vi "Scale and Checksum.vi"(0 "Raw Data":bool[](array[boolean])=[FALSE, FALSE, FALSE, FALSE, FALSE, FALSE, FALSE, FALSE, FALSE, FALSE, FALSE, FALSE, FALSE, FALSE, FALSE, FALSE, FALSE, FALSE, FALSE, FALSE, FALSE, FALSE, FALSE, FALSE, FALSE, FALSE, FALSE, FALSE, FALSE, FALSE, FALSE, FALSE, FALSE, FALSE, FALSE, FALSE, FALSE, FALSE, FALSE, FALSE]) -> (4 "Temperature (°C)":fxp<+,16,7> format="%.12g", 8 "Humidity (%)":fxp<+/-,18,8> format="%.13g", 15 "Valid?":bool)   [LabVIEW 2016, in "DHT22 (FPGA).lvlib"]
uses:
  DHT22 (FPGA).lvlib
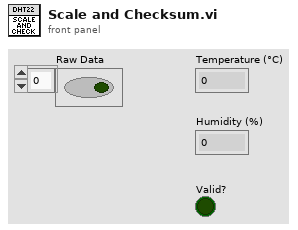
[diagram p1: front panel]
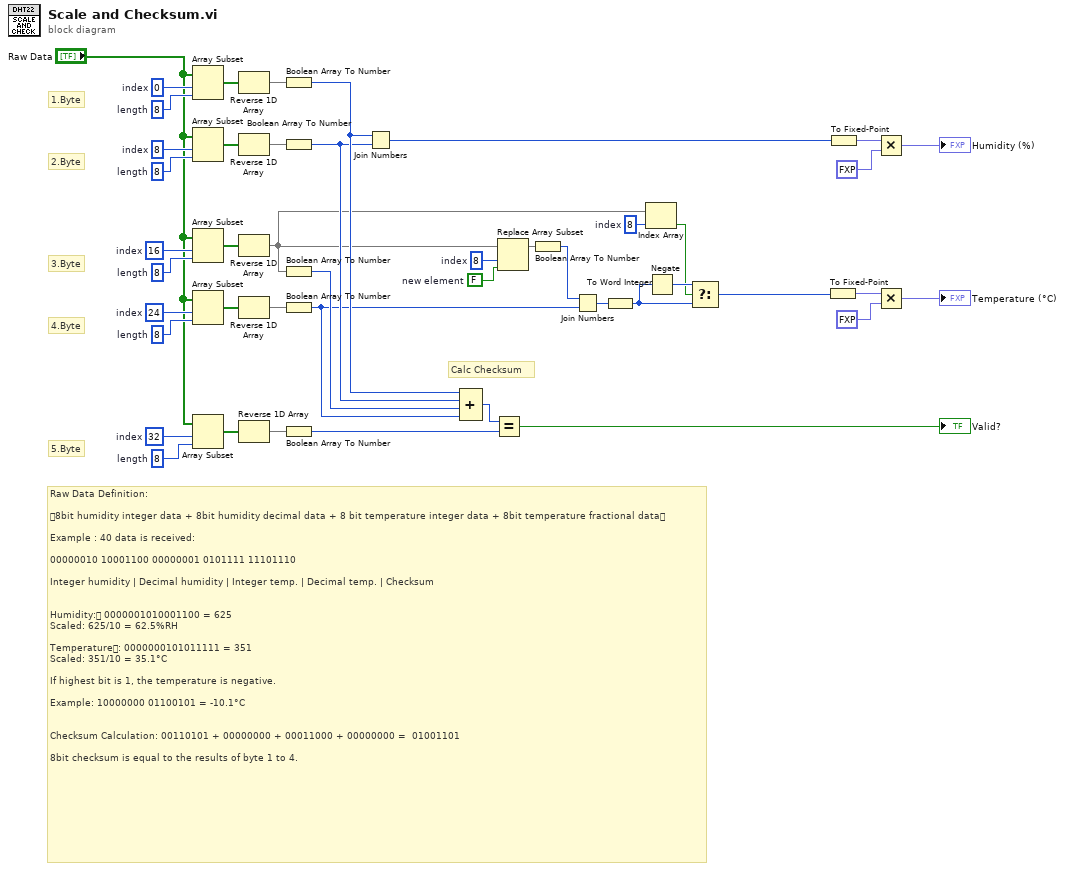
[diagram p0: block diagram]
diagram:
  w14 = 8  # index
  w15 = FALSE  # new element
  w13 = 8  # index
  w26 = 8  # length
  w27 = 24  # index
  w31 = 8  # length
  w30 = 8  # index
  w40 = 8  # length
  w41 = 32  # index
  w43 = 8  # length
  w42 = 16  # index
  w44 = 8  # length
  w45 = 0  # index
  # "Calc Checksum"
  # "4.Byte"
  # "2.Byte"
  # "5.Byte"
  # "3.Byte"
  # "1.Byte"
  # "Raw Data Definition:\n\n8bit humidity integer data + 8bit humidity decimal data + 8 bit temperature integer data + 8bit temperature fractional data\n\nExample : 40 data is received:\n\n00000010 10001100 00000001 0101111 11101110\n\nInteger humidity | Decimal humidity | Integer temp. | Decimal temp. | Checksum\n\n\nHumidity: 0000001010001100 = 625\nScaled: 625/10 = 62.5%RH\n\nTemperature: 0000000101011111 = 351\nScaled: 351/10 = 35.1°C\n\nIf highest bit is 1, the temperature is negative.\n\nExample: 10000000 01100101 = -10.1°C\n\n\nChecksum Calculation: 00110101 + 00000000 + 00011000 + 00000000 =  01001101\n\n8bit checksum is equal to the results of byte 1 to 4."
  n1 = Array Subset(array="Raw Data", index=w45, length=w44) -> (w39:bool[])
  n2 = Array Subset(array="Raw Data", index=w30, length=w31) -> (w32:bool[])
  n3 = Array Subset(array="Raw Data", index=w42, length=w43) -> (w37:bool[])
  n4 = Array Subset(array="Raw Data", index=w27, length=w26) -> (w28:bool[])
  n5 = Array Subset(array="Raw Data", index=w41, length=w40) -> (w36:bool[])
  n6 = Reverse 1D Array(array=w39) -> (reversed array=w38:bool[])
  n7 = Reverse 1D Array(array=w32) -> (reversed array=w29:bool[])
  n8 = Reverse 1D Array(array=w37) -> (reversed array=w12:bool[])
  n9 = Reverse 1D Array(array=w28) -> (reversed array=w10:bool[])
  n10 = Reverse 1D Array(array=w36) -> (reversed array=w35:bool[])
  n11 = Boolean Array To Number(Boolean array=w38) -> (number=w24:u8)
  n12 = Boolean Array To Number(Boolean array=w29) -> (number=w23:u8)
  n13 = Boolean Array To Number(Boolean array=w12) -> (number=w22:u8)
  n14 = Boolean Array To Number(Boolean array=w10) -> (number=w11:u8)
  n15 = Boolean Array To Number(Boolean array=w35) -> (number=w34:u8)
  n16 = Join Numbers(hi=w24, lo=w23) -> ((hi.lo)=w6:u16)
  n17 = Compound Arithmetic op=ADD(w24, w23, w22, w11) -> (w25:u8)
  n18 = Equal?(x=w25, y=w34) -> (x = y?=→"Valid?":bool)
  n19 = Replace Array Subset(array=w12, new element=w15, index=w14) -> (w16:bool[])
  n20 = Boolean Array To Number(Boolean array=w16) -> (number=w17:u8)
  n21 = Join Numbers(hi=w17, lo=w11) -> ((hi.lo)=w20:u16)
  n22 = To Word Integer(number=w20) -> (16bit integer=w21:i16)
  n23 = Index Array(array=w12, index=w13) -> (element=w18:bool)
  n24 = Negate(x=w21) -> (-x=w19:i16)
  n25 = Select(t=w19, s=w18, f=w21) -> (s? t:f=w3:i16)
  n26 = To Fixed-Point(number=w3) -> (fixed-point=w2:fxp<+/-,16,16>)  [unwired: 1 in]
  n27 = To Fixed-Point(number=w6) -> (fixed-point=w8:fxp<+,16,16>)  [unwired: 1 in]
  n28 = Multiply(x=w8, y=fxp<+/-,18,8> 0.099609375 ("x*y")) -> (x*y=→"Humidity (%)":fxp<+/-,18,8>)
  n29 = Multiply(x=w2, y=fxp<+/-,18,8> 0.099609375 ("x*y")) -> (x*y=→"Temperature (°C)":fxp<+,16,7>)
